vi "Add Property.vi"(8 "error in":errorcluster, 10 "Property Nodes":refnum<k20>[](array[refnum]), 11 "Item Ref in":refnum<data-value>) -> (0 "error out":errorcluster, 3 "Item Ref out":refnum<data-value>)   [LabVIEW 2024, in "Config File Parser.lvlib" / "Property.lvclass"]
uses:
  Property.lvclass
  Item/Item.lvclass
  Property.lvclass/Property.ctl
  <vilib>/xml/Close Reference(Node).vi
  <vilib>/xml/NI_XML.lvlib
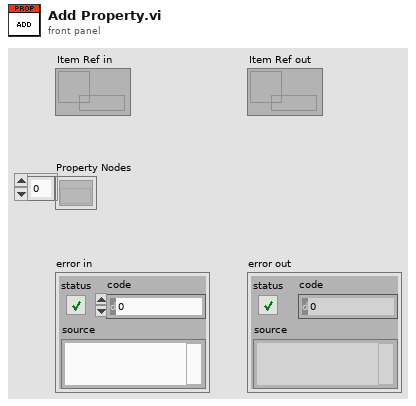
[diagram p1: front panel]
types:
  T1 = typedef "Config File Parser.lvlib/Property.lvclass/Property Type.ctl" = enum16{"Boolean", "Double", "String", "Path", "Dictionary", "DependentFile", "I16", "I32", "I64", "U16", "U32", "U64", "BooleanArray", "DoubleArray", "StringArray", "I16Array", "I32Array", "I64Array", "U16Array", "U32Array", "U64Array", "Variant"}
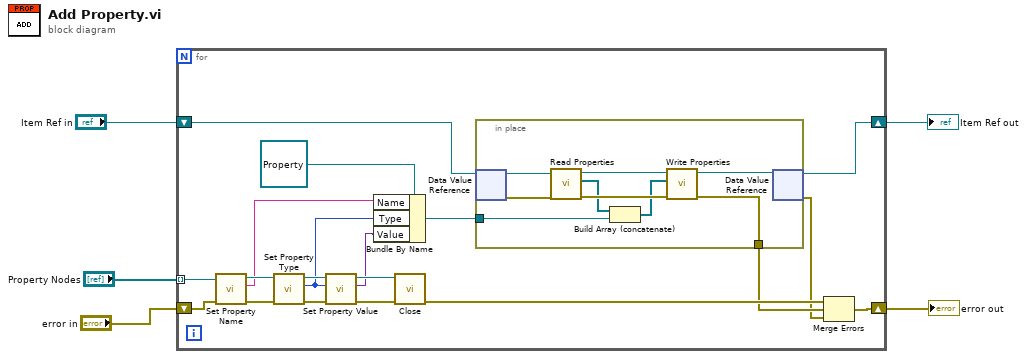
[diagram p0: block diagram]
diagram:
  n1 = for {
    tunnel: "Property Nodes" -> [w16] mode=indexing
    shift-right: [w6] -> w2
    shift-left: "Item Ref in" -> [w12]
    shift-right: [w18] -> w4
    shift-left: "error in" -> [w24]
    n2 = call "Set Property Name.vi"("error in"=w24, "Property Node in"=w16) -> ("error out"=w23:errorcluster, "Property Value"=w10:string, "Property Node out"=w15:refnum<k20>)  [unwired: 7 in]
    n3 = call "Set Property Type.vi"("error in"=w23, "Property Node"=w15) -> ("error out"=w22:errorcluster, "Property Type"=w9:T1, "Property Type Node"=w14:refnum<k20>)  [unwired: 7 in]
    n4 = call "Set Property Value.vi"("error in"=w22, "Property Type"=w9, "Property Type Node"=w14) -> ("error out"=w17:errorcluster, "Property Value"=w8:variant, "Property Type Node"=w13:refnum<k20>)  [unwired: 6 in]
    n5 = Bundle By Name(cluster=refnum<class "Property.lvclass"> refnum ("PropertyNode.lvclass"), "Name"=w10, "Type"=w9, "Value"=w8) -> (w7:refnum<class "Property.lvclass">)
    n6 = call-poly <vilib>:"Close.vi"("error in (no error)"=w17, "node"=w13) -> ("error out"=w21:errorcluster)  [unwired: 7 in]
    n7 = in-place "In Place Element Structure" {
      in-place-border: w7 -> [w26]
      in-place-border: [w31] -> w20
      n8 = in-place-dvr #1(w12) -> (w30:refnum<class "Item.lvclass">, w32:errorcluster)
      n9 = call-dynamic "Read Properties.vi"("error in (no error)"=w32, "Item in"=w30) -> ("error out"=w33:errorcluster, "Properties"=w27:refnum<class "Property.lvclass">[], "Item out"=w29:refnum<class "Item.lvclass">)  [unwired: 7 in]
      n10 = Build Array (concatenate)(w27, w26) -> (w25:refnum<class "Property.lvclass">[])
      n11 = call-dynamic "Write Properties.vi"("error in (no error)"=w33, "Properties"=w25, "Item in"=w29) -> ("error out"=w31:errorcluster, "Item out"=w28:refnum<class "Item.lvclass">)  [unwired: 7 in]
      n12 = in-place-dvr #1(w28) -> (w6:refnum<data-value>, w19:errorcluster)
    }
    n13 = Merge Errors(w21, w20, w19) -> (w18:errorcluster)
  }
  "error out" <- w4
  "Item Ref out" <- w2
